vi "Toggle_On_Press.vi"(1 "Boolean":bool) -> (0 "Boolean Out":bool)   [LabVIEW 2018]
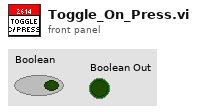
[diagram p1: front panel]
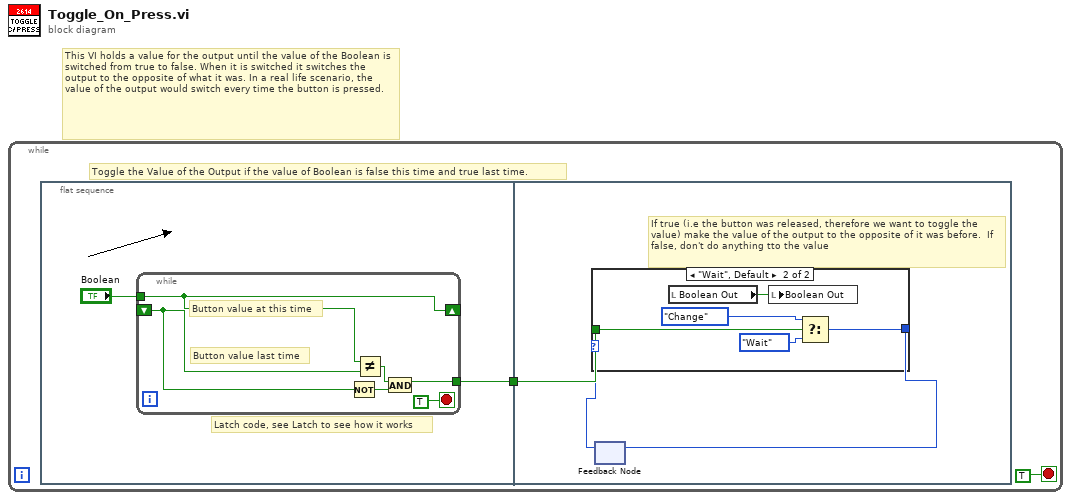
[diagram p0: block diagram]
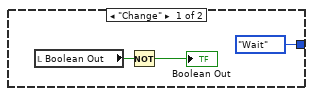
[diagram p2: hidden frame]
diagram:
  # "This VI holds a value for the output until the value of the Boolean is switched from true to false. When it is switched it switches the output to the opposite of what it was. In a real life scenario, the value of the output would switch every time the button is pressed."
  n1 = while {
    stop <- TRUE stop-if-true
    # "Toggle the Value of the Output if the value of Boolean is false this time and true last time."
    n2 = flat-sequence {
      tunnel: [w3] -> w1
      tunnel: w1 -> [w13]
      frame #0 {
        # "Latch code, see Latch to see how it works"
        n3 = while {
          tunnel: [w7] -> w3
          tunnel: "Boolean" -> [w10]
          shift-right: [w10] -> _
          shift-left: _ -> [w6]
          stop <- TRUE ("stop") stop-if-true
          # "Button value last time"
          # "Button value at this time"
          n4 = Not(x=w6) -> (.not. x?=w5:bool)
          n5 = Not Equal?(x=w10, y=w6) -> (x != y?=w8:bool)
          n6 = And(x=w8, y=w5) -> (x .and. y?=w7:bool)
        }
      }
      frame #1 {
        # "If true (i.e the button was released, therefore we want to toggle the value) make the value of the output to the opposite of it was before.  If false, don't do anything tto the value"
        n7 = feedback #1() -> (w11:enum16{"Change", "Wait"})  [unwired: 1 in]
        n8 = case shown="\"Wait\", Default" w11 {
          tunnel: w13 -> [_ w20]
          tunnel: [enum16{"Change", "Wait"}."Wait" w19] -> w12
          frame "Change" {
            n9 = local read "Boolean Out"() -> (w16:bool)
            n10 = Not(x=w16) -> (.not. x?=→"Boolean Out":bool)
          }
          frame "Wait", Default {
            n11 = local read "Boolean Out"() -> (w17:bool)
            n12 = local write "Boolean Out"(w17) -> ()
            n13 = Select(t=enum16{"Change", "Wait"}."Change", s=w20, f=enum16{"Change", "Wait"}."Wait") -> (s? t:f=w19:enum16{"Change", "Wait"})
          }
        }
        n14 = feedback-in #1(w12) -> ()
      }
    }
  }
